vi "asAcq_init.vi"(0 "reference":refnum<class "OSA.lvclass">, 5 "error in (no error)":errorcluster) -> (14 "duplicate reference":refnum<class "OSA.lvclass">, 19 "error out":errorcluster)   [LabVIEW 2010, in "OSA.lvclass"]
uses:
  OSA.lvclass
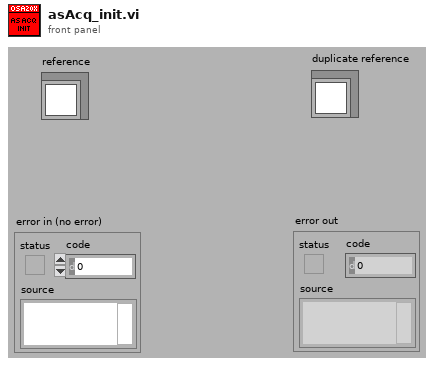
[diagram p1: front panel]
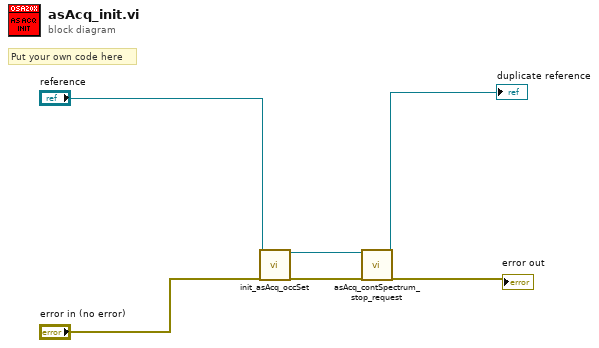
[diagram p0: block diagram]
diagram:
  # "Put your own code here"
  n1 = call "init_asAcq_occSet.vi"("reference"="reference", "error in (no error)"="error in (no error)") -> ("duplicate reference"=w4:refnum<class "OSA.lvclass">, "error out"=w3:errorcluster)  [unwired: 16 in]
  n2 = call "asAcq_contSpectrum_stop_request.vi"("reference"=w4, "error in (no error)"=w3) -> ("duplicate reference"=→"duplicate reference":refnum<class "OSA.lvclass">, "error out"=→"error out":errorcluster)  [unwired: 16 in]
